vi "Set Acquisition Configuration.vi"(8 "error in (no error)":errorcluster, 11 "CCDCamera in":refnum<class "Real Camera.lvclass">) -> (0 "error out":errorcluster, 3 "CCDCamera out":refnum<class "Real Camera.lvclass">)   [LabVIEW 2018, in "Real Camera.lvclass"]
doc: "Set the camera configuration\n\nThis function records the given operating parameters in the camera. However, the parameters will only bewritten if their last value is different from the most recent one."
uses:
  Real Camera.lvclass
panel:
  out "x != y? 2":T1
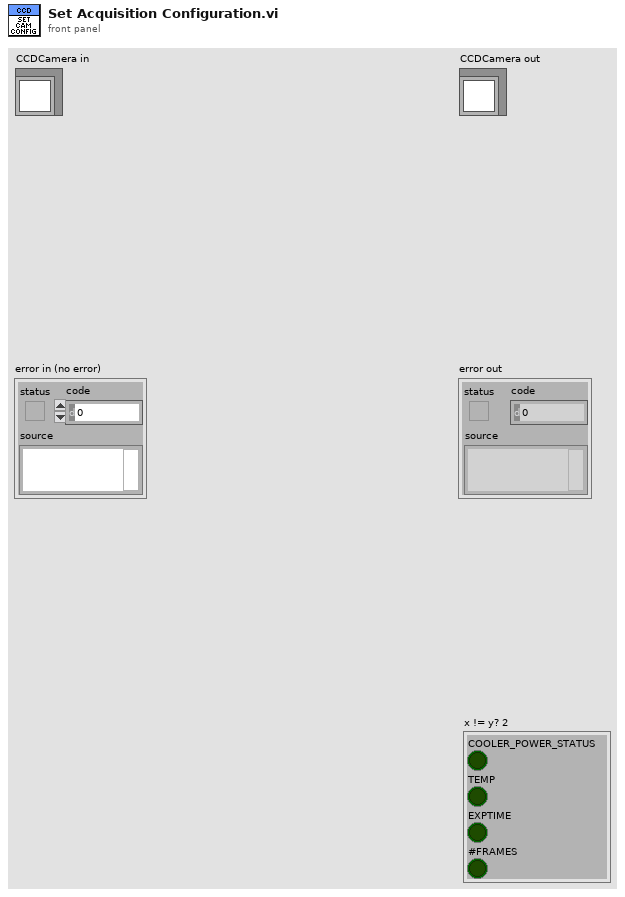
[diagram p1: front panel]
types:
  T1 = cluster{"COOLER_POWER_STATUS":bool, "TEMP":bool, "EXPTIME":bool, "#FRAMES":bool}
  T2 = cluster{"COOLER_POWER_STATUS":u16, "TEMP":i32, "EXPTIME":dbl, "#FRAMES":u32}
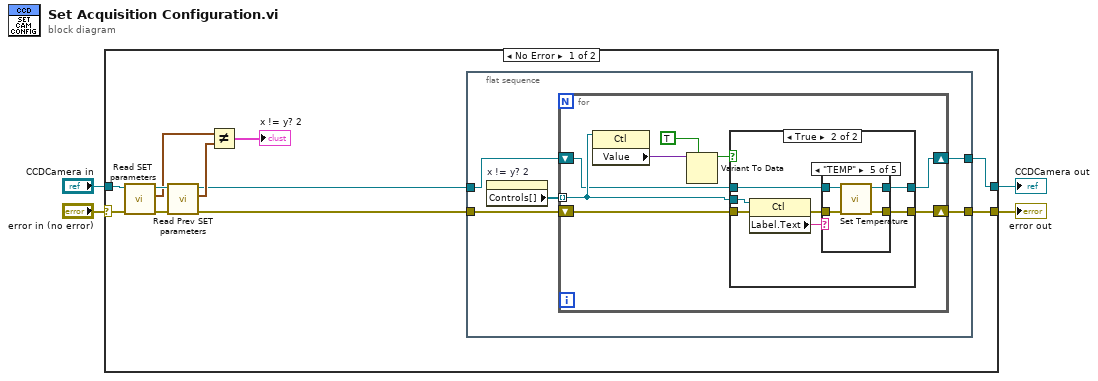
[diagram p0: block diagram]
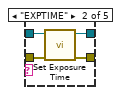
[diagram p4: hidden frame]
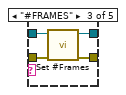
[diagram p5: hidden frame]
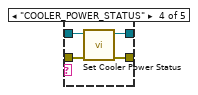
[diagram p6: hidden frame]
diagram:
  n1 = case shown="No Error" "error in (no error)" {
    selector: "error in (no error)" -> [w5 w57]
    tunnel: [w15 w57] -> w4
    tunnel: [w14 w56] -> w3
    tunnel: "CCDCamera in" -> [w6 w56]
    frame No Error {
      n2 = call-dynamic "Read SET parameters.vi"("error in (no error)"=w5, "Simulated_CCD_Camera in"=w6) -> ("error out"=w13:errorcluster, "New SET parameters"=w10:T2, "Simulated_CCD_Camera out"=w12:refnum<class "Real Camera.lvclass">)  [unwired: 7 in]
      n3 = call-dynamic "Read Prev SET parameters.vi"("error in (no error)"=w13, "Simulated_CCD_Camera in"=w12) -> ("error out"=w8:errorcluster, "Prev SET parameters"=w11:T2, "Simulated_CCD_Camera out"=w9:refnum<class "Real Camera.lvclass">)  [unwired: 7 in]
      n4 = Not Equal?(x=w10, y=w11) -> (x != y?=→"x != y? 2":T1)
      n5 = flat-sequence {
        tunnel: w8 -> [w16]
        tunnel: [w20] -> w15
        tunnel: w9 -> [w19]
        tunnel: [w18] -> w14
        frame #0 {
          n6 = property on="x != y? 2" class="Clust (strict)"() -> ("Controls[]"=w17:refnum<vi>[])  [unwired: 2 in, 2 out]
          n7 = for {
            tunnel: w17 -> [w27] mode=indexing
            shift-right: [w21] -> w20
            shift-left: w16 -> [w28]
            shift-right: [w22] -> w18
            shift-left: w19 -> [w23]
            n8 = property class="Ctl"(reference=w27) -> ("Value"=w26:variant)  [unwired: 1 in, 2 out]
            n9 = Variant To Data(type=TRUE, Variant=w26) -> (data=w24:bool)  [unwired: 1 in, 1 out]
            n10 = case shown="True" w24 {
              tunnel: w27 -> [_ w37]
              tunnel: [w30 w31] -> w21
              tunnel: w28 -> [w30 w35]
              tunnel: w23 -> [w29 w34]
              tunnel: [w29 w33] -> w22
              frame False {
              }
              frame True {
                n11 = property class="Ctl"(reference=w37, error in=w35) -> (error out=w32:errorcluster, "Label.Text"=w36:string)  [unwired: 1 out]
                n12 = case shown="\"TEMP\"" w36 {
                  tunnel: w34 -> [w39 w43 w46 w50 w55]
                  tunnel: [w39 w42 w47 w51 w54] -> w33
                  tunnel: w32 -> [w38 w41 w45 w49 w53]
                  tunnel: [w38 w40 w44 w48 w52] -> w31
                  frame "False", Default {
                  }
                  frame "EXPTIME" {
                    n13 = call-dynamic "Set Exposure Time.vi"("error in (no error)"=w41, "CCDCamera in"=w43) -> ("error out"=w40:errorcluster, "CCDCamera out"=w42:refnum<class "Real Camera.lvclass">)  [unwired: 8 in]
                  }
                  frame "#FRAMES" {
                    n14 = call-dynamic "Set #Frames.vi"("error in (no error)"=w45, "CCDCamera in"=w46) -> ("error out"=w44:errorcluster, "CCDCamera out"=w47:refnum<class "Real Camera.lvclass">)  [unwired: 8 in]
                  }
                  frame "COOLER_POWER_STATUS" {
                    n15 = call-dynamic "Set Cooler Power Status.vi"("error in (no error)"=w49, "CCDCamera in"=w50) -> ("error out"=w48:errorcluster, "CCDCamera out"=w51:refnum<class "Real Camera.lvclass">)  [unwired: 8 in]
                  }
                  frame "TEMP" {
                    n16 = call-dynamic "Set Temperature.vi"("error in (no error)"=w53, "CCDCamera in"=w55) -> ("error out"=w52:errorcluster, "CCDCamera out"=w54:refnum<class "Real Camera.lvclass">)  [unwired: 8 in]
                  }
                }
              }
            }
          }
        }
      }
    }
    frame Error {
    }
  }
  "error out" <- w4
  "CCDCamera out" <- w3
